vi "API Queue Manager.vi"(6 "Q_Select":T3, 8 "error in (no error)":errorcluster, 10 "Variant Data":variant, 11 "Command":string) -> (0 "error out":errorcluster, 3 "all X950 queues":T1)   [LabVIEW 2018]
uses:
  Command_Queue_Select.ctl
  All Module Queues.ctl
  Command_Queue_Ref.ctl
  Command Queue Cluster.ctl
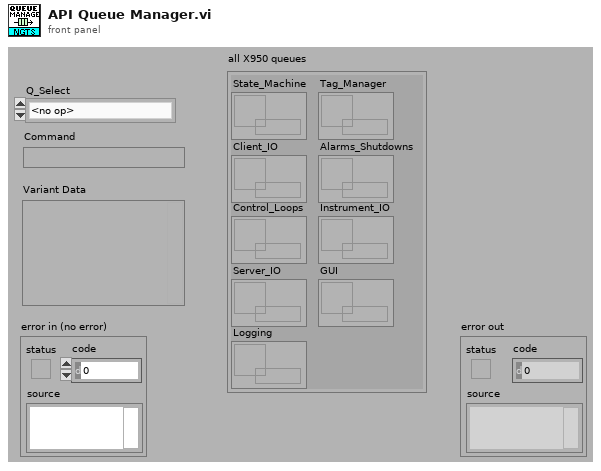
[diagram p1: front panel]
types:
  T1 = typedef "All Module Queues.ctl" = cluster{"State_Machine":T2, "Tag_Manager":T2, "Client_IO":T2, "Alarms_Shutdowns":T2, "Control_Loops":T2, "Instrument_IO":T2, "Server_IO":T2, "GUI":T2, "Logging":T2}
  T2 = typedef "Command_Queue_Ref.ctl" = refnum<queue>
  T3 = typedef "Command_Queue_Select.ctl" = enum16{"<no op>", "Destroy Queues", "Send -> State_Machine", "Send -> Client_IO", "Send -> Logging", "Send -> Instrument_IO", "Send -> Tag_Manager", "Send -> Alarms_Shutdowns", "Send -> Control_Loops", "Send -> Server_IO", "Send -> GUI"}
  T4 = cluster{"Command":string, "Variant Data":variant}
  T5 = typedef "Command Queue Cluster.ctl" = cluster{"Command":string, "Variant Data":variant}
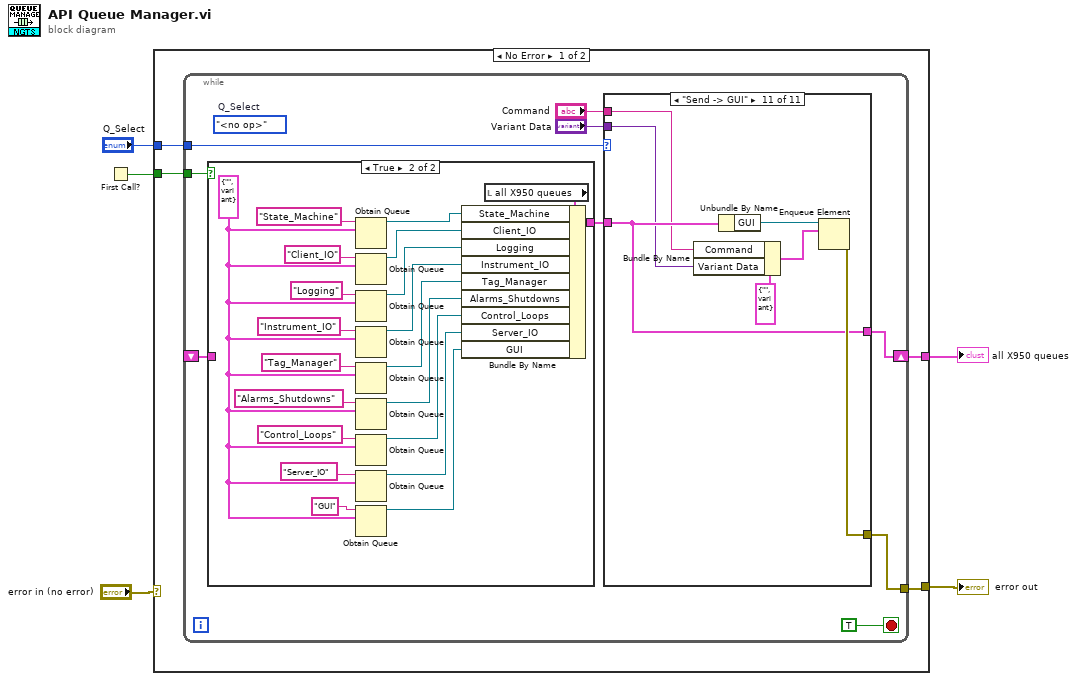
[diagram p0: block diagram]
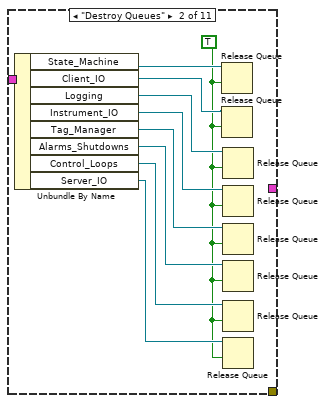
[diagram p3: hidden frame]
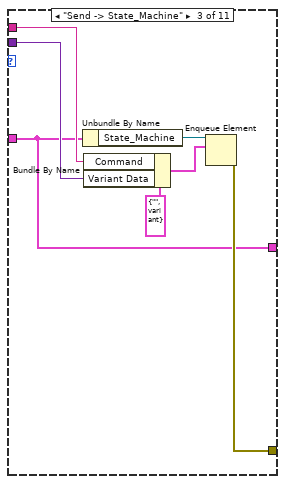
[diagram p4: hidden frame]
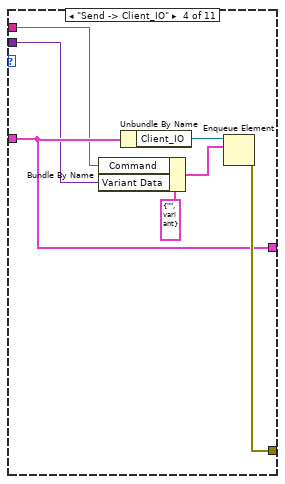
[diagram p5: hidden frame]
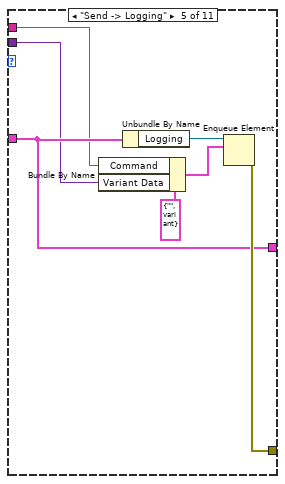
[diagram p6: hidden frame]
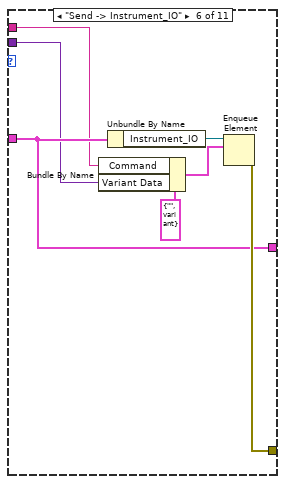
[diagram p7: hidden frame]
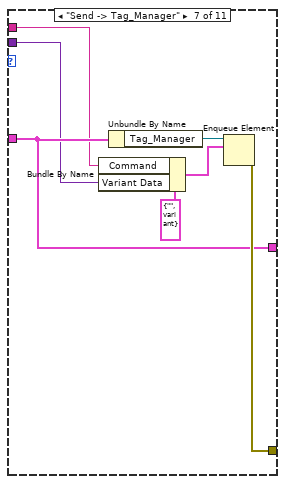
[diagram p8: hidden frame]
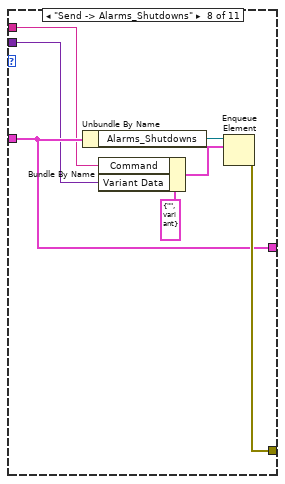
[diagram p9: hidden frame]
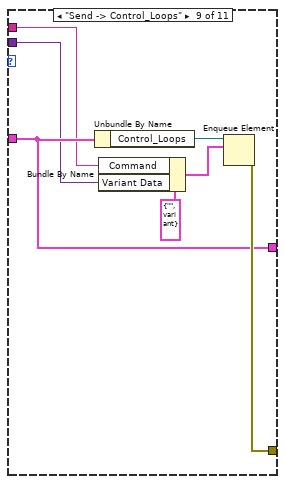
[diagram p10: hidden frame]
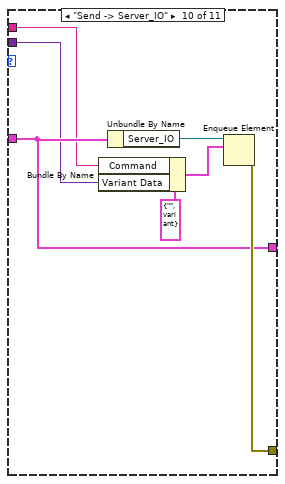
[diagram p11: hidden frame]
diagram:
  n1 = First Call?() -> (First Call?: T/F=w5:bool)
  n2 = case shown="No Error" "error in (no error)" {
    selector: "error in (no error)" -> [_ w115]
    tunnel: w5 -> [w9 _]
    tunnel: "Q_Select" -> [w8 _]
    tunnel: [w6 w115] -> w2
    tunnel: [w7 _] -> w1
    frame No Error {
      n3 = while {
        tunnel: w9 -> [w18]
        tunnel: w8 -> [w17]
        shift-right: [w15] -> w7
        shift-left: _ -> [w14]
        tunnel: [w11] -> w6
        stop <- TRUE stop-if-true
        (unwired) Command_Queue_Select."<no op>"  # Q_Select
        n4 = case shown="True" w18 {
          tunnel: [w93 w113] -> w16
          tunnel: w14 -> [w93 _]
          frame False {
          }
          frame True {
            w96 = T5 {"Command"="", "Variant Data"=variant} ("queue data")
            n5 = Obtain Queue(name (unnamed)="State_Machine", element data type=w96) -> (queue out=w112:refnum<queue>)  [unwired: 3 in, 2 out]
            n6 = Obtain Queue(name (unnamed)="Client_IO", element data type=w96) -> (queue out=w109:refnum<queue>)  [unwired: 3 in, 2 out]
            n7 = Obtain Queue(name (unnamed)="Logging", element data type=w96) -> (queue out=w107:refnum<queue>)  [unwired: 3 in, 2 out]
            n8 = Obtain Queue(name (unnamed)="Instrument_IO", element data type=w96) -> (queue out=w102:refnum<queue>)  [unwired: 3 in, 2 out]
            n9 = Obtain Queue(name (unnamed)="Tag_Manager", element data type=w96) -> (queue out=w101:refnum<queue>)  [unwired: 3 in, 2 out]
            n10 = Obtain Queue(name (unnamed)="Alarms_Shutdowns", element data type=w96) -> (queue out=w104:refnum<queue>)  [unwired: 3 in, 2 out]
            n11 = Obtain Queue(name (unnamed)="Control_Loops", element data type=w96) -> (queue out=w99:refnum<queue>)  [unwired: 3 in, 2 out]
            n12 = Obtain Queue(name (unnamed)="Server_IO", element data type=w96) -> (queue out=w97:refnum<queue>)  [unwired: 3 in, 2 out]
            n13 = Obtain Queue(name (unnamed)="GUI", element data type=w96) -> (queue out=w94:refnum<queue>)  [unwired: 3 in, 2 out]
            n14 = local read "all X950 queues"() -> (w111:T1)
            n15 = Bundle By Name(cluster=w111, "State_Machine"=w112, "Client_IO"=w109, "Logging"=w107, "Instrument_IO"=w102, "Tag_Manager"=w101, "Alarms_Shutdowns"=w104, "Control_Loops"=w99, "Server_IO"=w97, "GUI"=w94) -> (w113:T1)
          }
        }
        n16 = case shown="\"Send -> GUI\"" w17 {
          tunnel: [w19 _ w30 w42 w49 w56 w63 w70 w77 w84 w91] -> w15
          tunnel: w16 -> [w19 w29 w30 w42 w49 w56 w63 w70 w77 w84 w91]
          tunnel: "Command" -> [_ _ w35 w39 w46 w53 w60 w67 w74 w81 w88]
          tunnel: "Variant Data" -> [_ _ w34 w38 w45 w52 w59 w66 w73 w80 w87]
          tunnel: [_ _ w31 w43 w50 w57 w64 w71 w78 w85 w92] -> w11
          frame "<no op>" {
          }
          frame "Destroy Queues" {
            w20 = TRUE ("force destroy? (F)")
            n17 = Unbundle By Name(w29) -> ("State_Machine"=w28:T2, "Client_IO"=w27:T2, "Logging"=w26:T2, "Instrument_IO"=w23:T2, "Tag_Manager"=w25:T2, "Alarms_Shutdowns"=w24:T2, "Control_Loops"=w22:T2, "Server_IO"=w21:T2)
            n18 = Release Queue(queue=w28, force destroy? (F)=w20) -> ()  [unwired: 1 in, 3 out]
            n19 = Release Queue(queue=w27, force destroy? (F)=w20) -> ()  [unwired: 1 in, 3 out]
            n20 = Release Queue(queue=w26, force destroy? (F)=w20) -> ()  [unwired: 1 in, 3 out]
            n21 = Release Queue(queue=w23, force destroy? (F)=w20) -> ()  [unwired: 1 in, 3 out]
            n22 = Release Queue(queue=w25, force destroy? (F)=w20) -> ()  [unwired: 1 in, 3 out]
            n23 = Release Queue(queue=w24, force destroy? (F)=w20) -> ()  [unwired: 1 in, 3 out]
            n24 = Release Queue(queue=w22, force destroy? (F)=w20) -> ()  [unwired: 1 in, 3 out]
            n25 = Release Queue(queue=w21, force destroy? (F)=w20) -> ()  [unwired: 1 in, 3 out]
          }
          frame "Send -> State_Machine" {
            n26 = Unbundle By Name(w30) -> ("State_Machine"=w33:T2)
            n27 = Bundle By Name(cluster=T4 {"Command"="", "Variant Data"=variant} ("main window queue datatype"), "Command"=w35, "Variant Data"=w34) -> (w32:T4)
            n28 = Enqueue Element(queue=w33, element=w32) -> (error out=w31:errorcluster)  [unwired: 2 in, 2 out]
          }
          frame "Send -> Client_IO" {
            n29 = Bundle By Name(cluster=T4 {"Command"="", "Variant Data"=variant} ("main window queue datatype"), "Command"=w39, "Variant Data"=w38) -> (w37:T4)
            n30 = Unbundle By Name(w42) -> ("Client_IO"=w41:T2)
            n31 = Enqueue Element(queue=w41, element=w37) -> (error out=w43:errorcluster)  [unwired: 2 in, 2 out]
          }
          frame "Send -> Logging" {
            n32 = Bundle By Name(cluster=T4 {"Command"="", "Variant Data"=variant} ("main window queue datatype"), "Command"=w46, "Variant Data"=w45) -> (w44:T4)
            n33 = Unbundle By Name(w49) -> ("Logging"=w48:T2)
            n34 = Enqueue Element(queue=w48, element=w44) -> (error out=w50:errorcluster)  [unwired: 2 in, 2 out]
          }
          frame "Send -> Instrument_IO" {
            n35 = Bundle By Name(cluster=T4 {"Command"="", "Variant Data"=variant} ("main window queue datatype"), "Command"=w53, "Variant Data"=w52) -> (w51:T4)
            n36 = Unbundle By Name(w56) -> ("Instrument_IO"=w55:T2)
            n37 = Enqueue Element(queue=w55, element=w51) -> (error out=w57:errorcluster)  [unwired: 2 in, 2 out]
          }
          frame "Send -> Tag_Manager" {
            n38 = Bundle By Name(cluster=T4 {"Command"="", "Variant Data"=variant} ("main window queue datatype"), "Command"=w60, "Variant Data"=w59) -> (w58:T4)
            n39 = Unbundle By Name(w63) -> ("Tag_Manager"=w62:T2)
            n40 = Enqueue Element(queue=w62, element=w58) -> (error out=w64:errorcluster)  [unwired: 2 in, 2 out]
          }
          frame "Send -> Alarms_Shutdowns" {
            n41 = Unbundle By Name(w70) -> ("Alarms_Shutdowns"=w69:T2)
            n42 = Bundle By Name(cluster=T4 {"Command"="", "Variant Data"=variant} ("main window queue datatype"), "Command"=w67, "Variant Data"=w66) -> (w65:T4)
            n43 = Enqueue Element(queue=w69, element=w65) -> (error out=w71:errorcluster)  [unwired: 2 in, 2 out]
          }
          frame "Send -> Control_Loops" {
            n44 = Unbundle By Name(w77) -> ("Control_Loops"=w76:T2)
            n45 = Bundle By Name(cluster=T4 {"Command"="", "Variant Data"=variant} ("main window queue datatype"), "Command"=w74, "Variant Data"=w73) -> (w72:T4)
            n46 = Enqueue Element(queue=w76, element=w72) -> (error out=w78:errorcluster)  [unwired: 2 in, 2 out]
          }
          frame "Send -> Server_IO" {
            n47 = Bundle By Name(cluster=T4 {"Command"="", "Variant Data"=variant} ("main window queue datatype"), "Command"=w81, "Variant Data"=w80) -> (w79:T4)
            n48 = Unbundle By Name(w84) -> ("Server_IO"=w83:T2)
            n49 = Enqueue Element(queue=w83, element=w79) -> (error out=w85:errorcluster)  [unwired: 2 in, 2 out]
          }
          frame "Send -> GUI" {
            n50 = Bundle By Name(cluster=T4 {"Command"="", "Variant Data"=variant} ("main window queue datatype"), "Command"=w88, "Variant Data"=w87) -> (w86:T4)
            n51 = Unbundle By Name(w91) -> ("GUI"=w90:T2)
            n52 = Enqueue Element(queue=w90, element=w86) -> (error out=w92:errorcluster)  [unwired: 2 in, 2 out]
          }
        }
      }
    }
    frame Error {
    }
  }
  "error out" <- w2
  "all X950 queues" <- w1
